vi "Initialize.vi"(0 "Manual Cal Standard in":refnum<class "Cal Standard.lvclass">, 11 "error in (no error)":errorcluster) -> (4 "Manual Cal Standard out":refnum<class "Cal Standard.lvclass">, 6 "Found":bool, 15 "error out":errorcluster)   [LabVIEW 2023, in "Manual Cal Standard.lvlib" / "Cal Standard.lvclass"]
uses:
  Cal Standard.lvclass
  C:/srd-semi-rfcal-software/AuxTools/STSRFFixtureCharactUtility/Source/Code Modules/Fixture/Instruments/Cal Standard/Cal Standard Base/Cal Standard Base.lvclass
  Instruments/Cal Standard/Type Definitions/One-Port Cal Standard.ctl
  Instruments/Cal Standard/Type Definitions/One-Port Charact Data.ctl
  Instruments/Cal Standard/Type Definitions/Standard Type.ctl
  Instruments/Cal Standard/Cal Standard Base/Cal Standard Base.lvclass/Cal Standard Base.ctl
  Instruments/Cal Standard/Cal Standard Base/Properties/Write Instrument Info.vi
  Instruments/Cal Standard/Cal Standard Base/Properties/Write Path Connection Map.vi
  Utilities/Setting Keys.vi
  Dependencies/HFNetworkAnalysis/Support VIs/Read SnP File (S1P).vi
  Instruments/Cal Standard/Cal Standard Base/Properties/Write One-Port Cal Standards.vi
  Instruments/RFFixtureCharact.Instruments.lvlib
  Common/RFCalAndFixtureCharact.Common.lvlib
  Dependencies/HFNetworkAnalysis/NI_HFNetworkAnalysis.lvlib
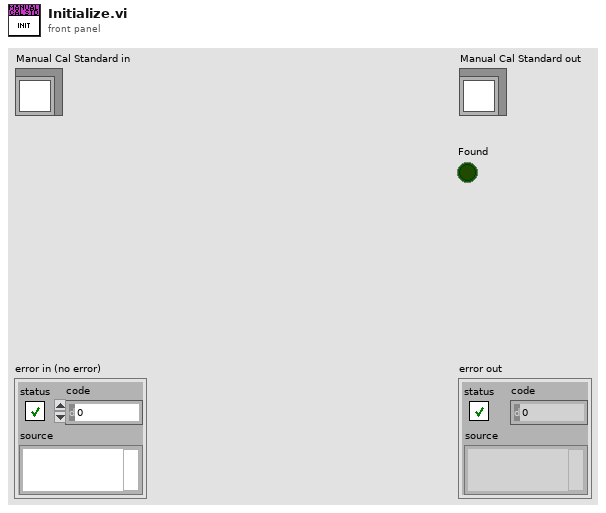
[diagram p1: front panel]
types:
  T1 = typedef "RFFixtureCharact.Instruments.lvlib/One-Port Cal Standard.ctl" = cluster{"Port Name":string, "Charact Data":T2[]}
  T2 = typedef "RFFixtureCharact.Instruments.lvlib/One-Port Charact Data.ctl" = cluster{"Standard Type":T3, "Frequencies":dbl[], "S11":cdb[]}
  T3 = typedef "RFFixtureCharact.Instruments.lvlib/Standard Type.ctl" = enum16{"Short", "Open", "Load"}
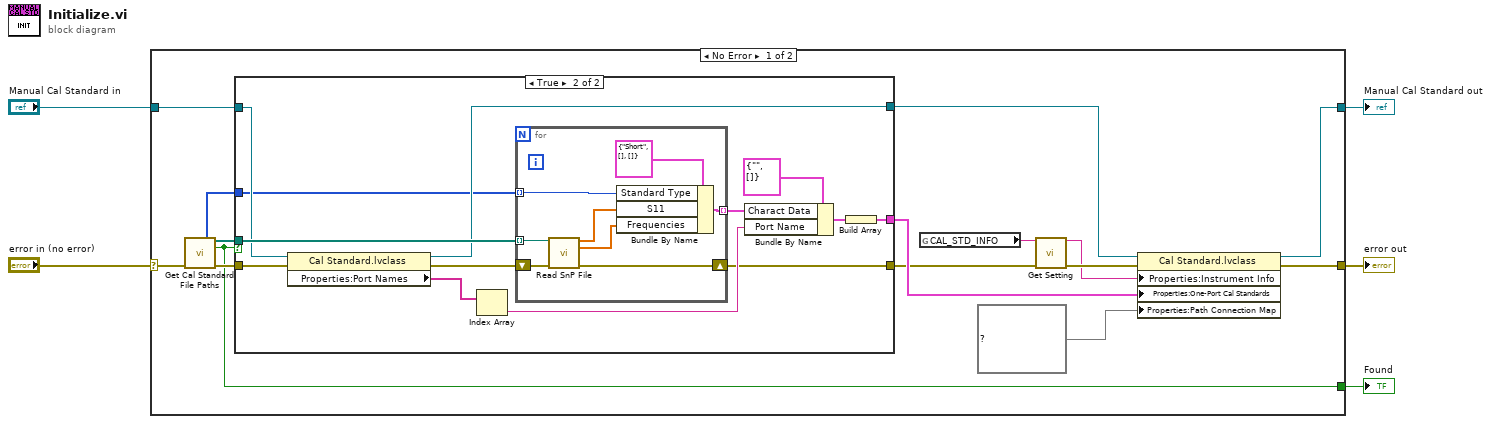
[diagram p0: block diagram]
diagram:
  n1 = case shown="No Error" "error in (no error)" {
    selector: "error in (no error)" -> [w14 w45]
    tunnel: [w20 w45] -> w1
    tunnel: [w19 w44] -> w4
    tunnel: "Manual Cal Standard in" -> [w11 w44]
    tunnel: [w7 _] -> w3
    frame No Error {
      n2 = call "Get Cal Standard File Paths.vi"("error in (no error)"=w14) -> ("Cal Standard Types"=w6:T3[], "Cal Standard File Paths"=w13:path[], "Found"=w7:bool, "error out"=w12:errorcluster)  [unwired: 11 in]
      n3 = case shown="True" w7 {
        tunnel: w13 -> [_ w35]
        tunnel: w12 -> [w22 w34]
        tunnel: w11 -> [w21 w32]
        tunnel: [_ w26] -> w10
        tunnel: [w22 w25] -> w9
        tunnel: [w21 w24] -> w8
        tunnel: w6 -> [_ w23]
        frame False {
        }
        frame True {
          n4 = property class="Cal Standard.lvclass"(reference=w32, error in=w34) -> (reference out=w24:refnum<class "Cal Standard.lvclass">, error out=w33:errorcluster, "Properties:Port Names"=w31:string[])
          n5 = Index Array(array=w31) -> (element=w28:string)  [unwired: 1 in]
          n6 = for {
            tunnel: w35 -> [w42] mode=indexing
            shift-right: [w37] -> w25
            shift-left: w33 -> [w43]
            tunnel: w23 -> [w40] mode=indexing
            tunnel: [w36] -> w29 mode=indexing
            n7 = call-poly "Read SnP File.vi"("S1P File Path"=w42, "Error In"=w43) -> ("S-parameters"=w39:cdb[], "Frequencies (Hz)"=w38:dbl[], "Error Out"=w37:errorcluster)  [unwired: 10 in, 1 out]
            n8 = Bundle By Name(cluster=T2 {"Standard Type"=enum."Short", "Frequencies"=[], "S11"=[]} ("Charact Data"), "Standard Type"=w40, "S11"=w39, "Frequencies"=w38) -> (w36:T2)
          }
          n9 = Bundle By Name(cluster=T1 {"Port Name"="", "Charact Data"=[]} ("One-Port Cal Standard"), "Charact Data"=w29, "Port Name"=w28) -> (w27:T1)
          n10 = Build Array(w27) -> (w26:T1[])
        }
      }
      n11 = global read "Setting Keys.vi" "CAL_STD_INFO"() -> (w16:string)
      n12 = call "Get Setting.vi"("Setting name"=w16, "error in (no error)"=w9) -> ("Setting value out"=w15:string, "error out"=w17:errorcluster)  [unwired: 11 in, 1 out]
      n13 = property class="Cal Standard.lvclass"(reference=w8, error in=w17, "Properties:Instrument Info"=w15, "Properties:One-Port Cal Standards"=w10, "Properties:Path Connection Map"=map{string, string[]} {} ("Path Connection Map")) -> (reference out=w19:refnum<class "Cal Standard.lvclass">, error out=w20:errorcluster)
    }
    frame Error {
    }
  }
  "error out" <- w1
  "Manual Cal Standard out" <- w4
  "Found" <- w3
